vi "launch core.vi"(5 "execution system":T1, 7 "thread pool in":refnum<class "thread pool.lvclass">, 8 "error in (no error)":errorcluster, 9 "queue size":i32, 11 "communicator in":refnum<class "communicator.lvclass">) -> (0 "error out":errorcluster, 1 "timed out?":bool, 3 "communicator out":refnum<class "communicator.lvclass">)   [LabVIEW 2015, in "communicator manager.lvlib"]
uses:
  communicator manager.lvlib
  communicator/communicator.lvclass
  taskpool/dispatcher/execution system.ctl
  taskpool/dispatcher/thread pool.lvclass
  communicator task/communicator task.lvclass
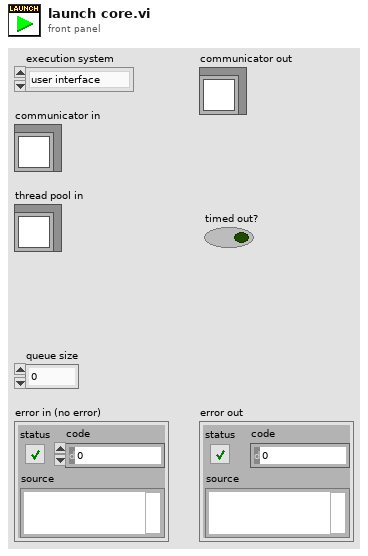
[diagram p1: front panel]
types:
  T1 = typedef "thread pool.lvclass/execution system.ctl" = enum32{"user interface", "standard", "instrument i/o", "data acquisition", "other 1", "other 2"}
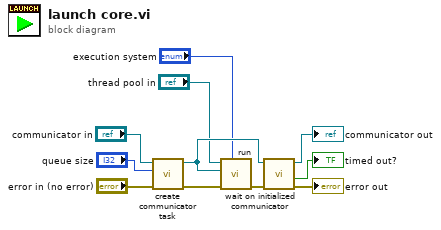
[diagram p0: block diagram]
diagram:
  n1 = call "create communicator task.vi"("error in"="error in (no error)", "queue size (1,10000)"="queue size", "communicator"="communicator in") -> ("error out"=w3:errorcluster, "communicator task out"=w8:refnum<class "communicator task.lvclass">)  [unwired: 7 in]
  n2 = call "run.vi"("execution system"="execution system", "error in"=w3, "task"=w8, "thread pool in"="thread pool in") -> ("error out"=w7:errorcluster)  [unwired: 6 in, 1 out]
  n3 = call "wait on initialized communicator.vi"("error in"=w7, "communicator task in"=w8) -> ("error out"=→"error out":errorcluster, "timed out?"=→"timed out?":bool, "initialized communicator"=→"communicator out":refnum<class "communicator.lvclass">)  [unwired: 7 in]
